vi "PWM_Count_11.vi"() -> ()   [LabVIEW 2019]
uses:
  <vilib>/rvi/Emulation/niFpgaGetClockAttributes.vi
  <vilib>/rvi/Emulation/niFpgaSctlEmulationGetInTimedLoop.vi
  <vilib>/rvi/Emulation/niFpgaEmulationReportErrorSimple.vi
  <vilib>/rvi/eio/common/nirviEmuTemplateMethod_errors.vi
  <vilib>/rvi/Emulation/niFpgaCriticalErrorInLSC.vi
  <vilib>/eio/EIONode/EIONode.xnode
panel:
  out "波形图表":sgl(graph)
  out "x-y":sgl
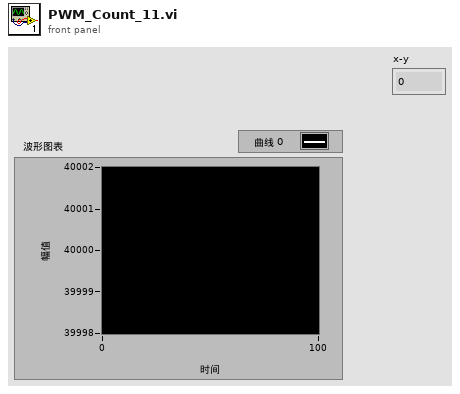
[diagram p1: front panel]
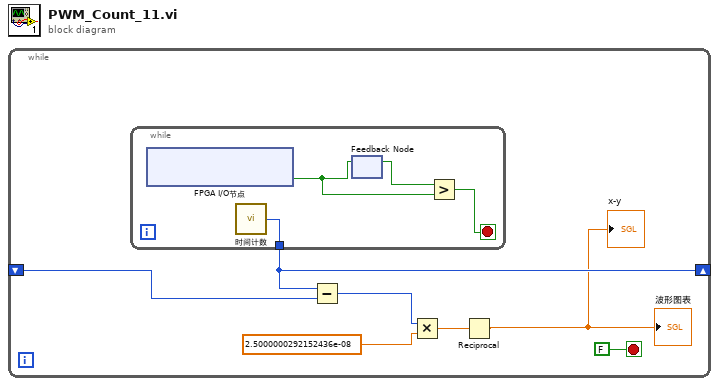
[diagram p0: block diagram]
diagram:
  n1 = while {
    shift-right: [w6] -> _
    shift-left: _ -> [w5]
    stop <- FALSE stop-if-true
    n2 = while {
      tunnel: [w8] -> w6
      stop <- w9 stop-if-true
      n3 = xnode "FPGA I/O节点"() -> ("ConnectorB/DIO0"=w10:bool)  [unwired: 1 in, 1 out]
      n4 = call "时间计数"() -> ("Tick Count(Ticks)"=w8:u32)
      n5 = feedback #1() -> (w11:bool)  [unwired: 1 in]
      n6 = feedback-in #1(w10) -> ()
      n7 = Greater?(x=w11, y=w10) -> (0:w9:bool)
    }
    n8 = Subtract(x=w6, y=w5) -> (x-y=w2:u32)
    n9 = Multiply(x=w2, y=sgl 2.5e-08) -> (x*y=w3:sgl)
    n10 = Reciprocal(x=w3) -> (1/x=→"x-y" →"波形图表":sgl)
  }
